vi "SR830_Get.vi"(8 "Error In":errorcluster caption="错误输入", 10 "数据长度":dbl, 11 "VISA 输入":refnum<visa-resource-name>="GPIB0::7::INSTR") -> (0 "Error Out":errorcluster caption="错误输出", 2 "Channel 2":sgl[](array[numeric]), 3 "Channel 1":sgl[](array[numeric]))   [LabVIEW 2020]
uses:
  lib/SR830/Public/Data/Read (Multiple Points).vi
  lib/SR830/SR830.lvlib
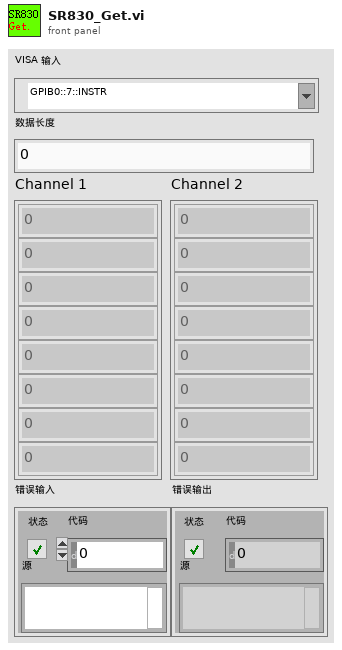
[diagram p1: front panel]
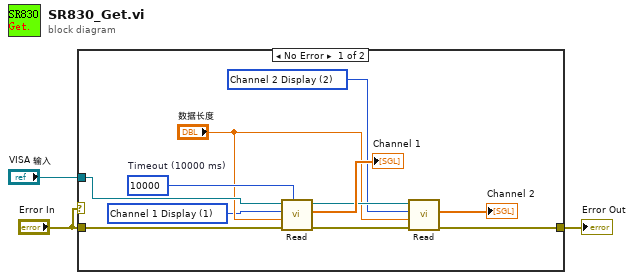
[diagram p0: block diagram]
diagram:
  n1 = case shown="No Error" "Error In" {
    tunnel: "Error In" -> [w13 w15]
    tunnel: [w9 w15] -> w2
    tunnel: "VISA 输入" -> [w12 _]
    frame No Error {
      w4 = u16 1 items=["Channel 1 Display"=1, "Channel 2 Display"=2] ("Channel (1: Channel 1 Display)")
      w5 = u16 2 items=["Channel 1 Display"=1, "Channel 2 Display"=2] ("Channel (1: Channel 1 Display)")
      w14 = u32 10000  # Timeout (10000 ms)
      n2 = call-poly "Read.vi"("Maximum Time (10000 ms)"=w14, "error in (no error)"=w13, "Number of Points (100)"="数据长度", "Channel (1: Channel 1 Display)"=w4, "VISA resource name"=w12) -> ("error out"=w10:errorcluster, "Measurements"=→"Channel 1":sgl[], "VISA resource name out"=w7:refnum<visa-resource-name>)  [unwired: 4 in]
      n3 = call-poly "Read.vi"("error in (no error)"=w10, "Number of Points (100)"="数据长度", "Channel (1: Channel 1 Display)"=w5, "VISA resource name"=w7) -> ("error out"=w9:errorcluster, "Measurements"=→"Channel 2":sgl[])  [unwired: 5 in, 1 out]
    }
    frame Error {
    }
  }
  "Error Out" <- w2
